vi "Reconfigure.vi"(8 "error in (no error)":errorcluster, 10 "navX - Interface Update in":refnum<class "navX - Interface.lvclass">, 11 "navX - SERIAL in":refnum<class "navX - SERIAL.lvclass">) -> (0 "error out":errorcluster, 3 "navX - SERIAL out":refnum<class "navX - SERIAL.lvclass">)   [LabVIEW 2015, in "navX Library v3.lvlib" / "navX - SERIAL.lvclass"]
uses:
  navX - SERIAL.lvclass
  navX - Interface/navX - Interface.lvclass
  navX - SERIAL.lvclass/navX - SERIAL.ctl
  navX - Interface/Notifications/Send Notification.vi
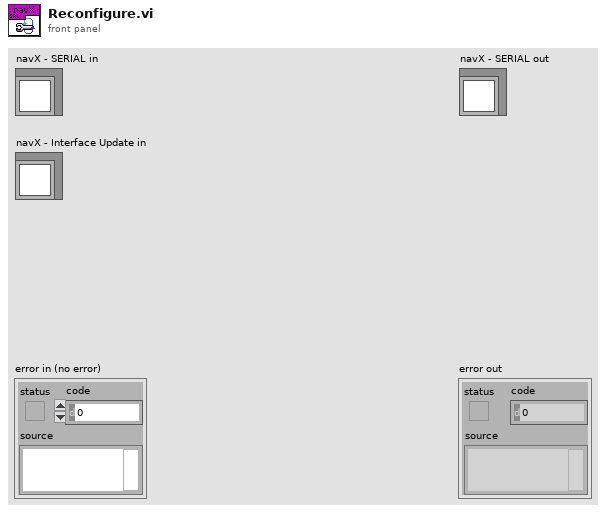
[diagram p1: front panel]
types:
  T1 = typedef "navX Library v3.lvlib/navX - SERIAL.lvclass/Protocol.ctl" = enum16{"YRPH", "Quaterinons", "Gyro/Raw", "AHRS", "AHRSAndPositioning"}
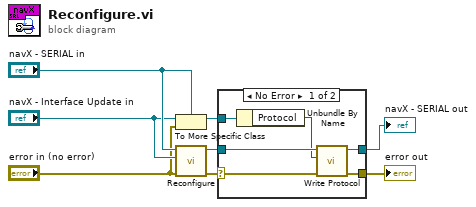
[diagram p0: block diagram]
diagram:
  n1 = To More Specific Class(target class="navX - SERIAL in", reference="navX - Interface Update in", error in="error in (no error)") -> (specific class reference=w3:refnum<class "navX - SERIAL.lvclass">)  [unwired: 1 out]
  n2 = call-parent "Reconfigure.vi"("error in (no error)"="error in (no error)", "navX - Interface Update in"="navX - Interface Update in", "navX - Interface in"="navX - SERIAL in") -> ("error out"=w8:errorcluster, "navX - Interface out"=w6:refnum<class "navX - SERIAL.lvclass">)  [unwired: 7 in]
  n3 = case shown="No Error" w8 {
    selector: w8 -> [w10 w16]
    tunnel: [w12 w16] -> w7
    tunnel: [w13 w15] -> w5
    tunnel: w6 -> [w14 w15]
    tunnel: w3 -> [w11 _]
    frame No Error {
      n4 = Unbundle By Name(w11) -> ("Protocol"=w9:T1)
      n5 = call "Write Protocol.vi"("error in (no error)"=w10, "Protocol"=w9, "navX - SERIAL in"=w14) -> ("error out"=w12:errorcluster, "navX - SERIAL out"=w13:refnum<class "navX - SERIAL.lvclass">)  [unwired: 7 in]
    }
    frame Error {
    }
  }
  "error out" <- w7
  "navX - SERIAL out" <- w5
